vi "Main Dialog.vi"(11 "Process Path":path) -> ()   [LabVIEW 2020, in "Method Generation.lvlib" / "New API VI Dialog.lvclass"]
uses:
  New API VI Dialog.lvclass
  New API VI Dialog.lvclass/New API VI Dialog.ctl
  API VI Generator/API VI Generator.lvclass
panel:
  in  "Highlight changes?":bool=TRUE
  in  "Commit":bool
  in  "Cancel":bool
  in  "API Message":string
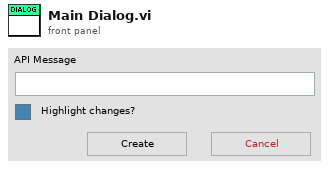
[diagram p1: front panel]
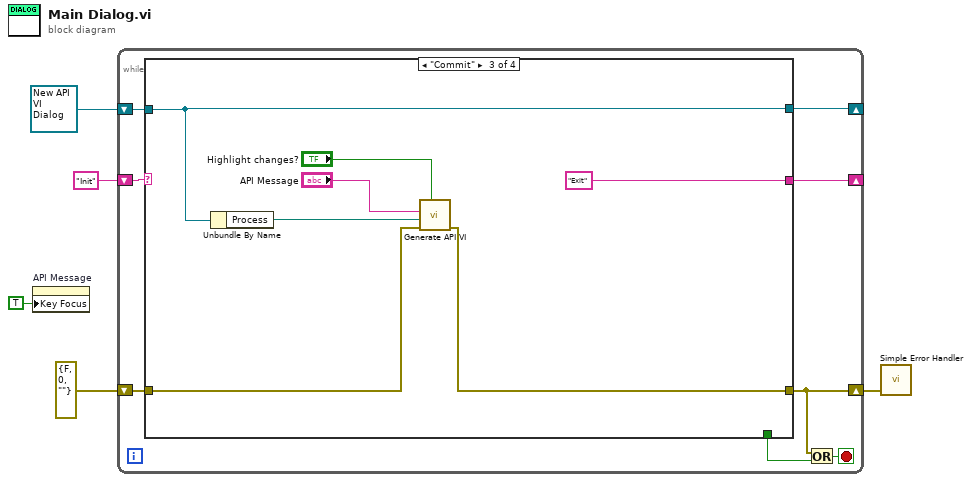
[diagram p0: block diagram]
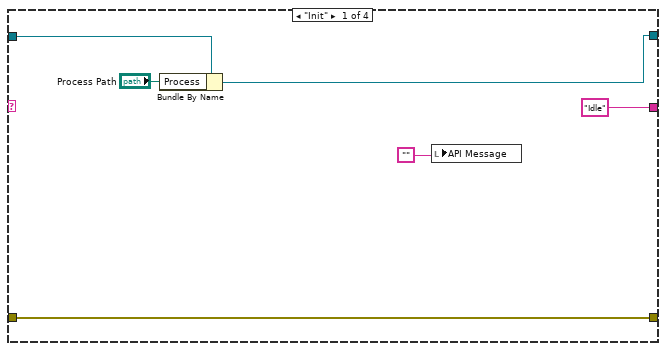
[diagram p2: hidden frame]
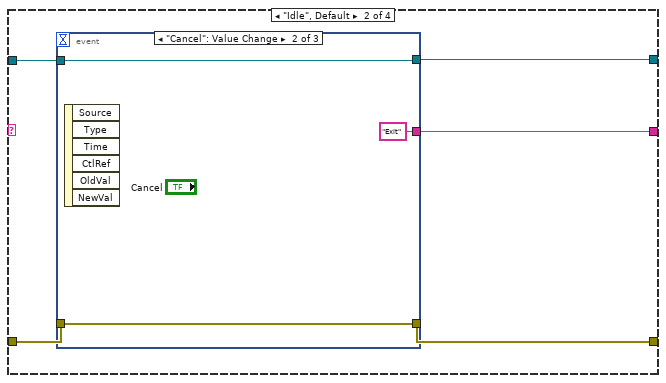
[diagram p3: hidden frame]
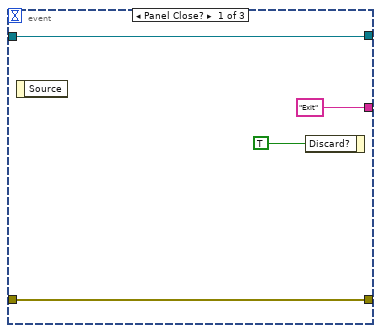
[diagram p4: hidden frame]
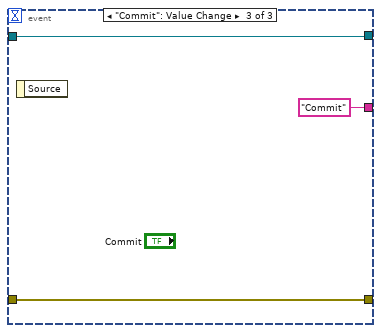
[diagram p5: hidden frame]
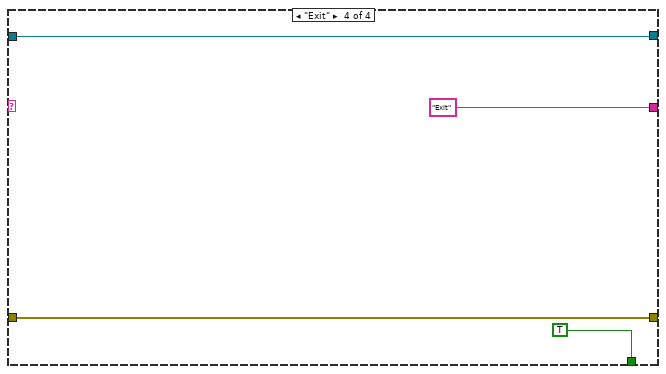
[diagram p6: hidden frame]
diagram:
  n1 = property on="API Message" class="Str"("Key Focus"=TRUE) -> ()  [unwired: 2 in, 2 out]
  n2 = while {
    shift-right: [w10] -> _
    shift-left: refnum<class "New API VI Dialog.lvclass"> refnum ("Method Generation.lvlib:New Getter Dialog.lvclass") -> [w11]
    shift-right: [w6] -> w2
    shift-left: errorcluster {"status"=FALSE, "code"=0, "source"=""} ("error in (no error)") -> [w12]
    shift-right: [w9] -> _
    shift-left: "Init" -> [w13]
    stop <- w7 stop-if-true
    n3 = case shown="\"Commit\"" w13 {
      tunnel: [w16 w24 w38 w44] -> w6
      tunnel: w12 -> [w16 w23 w37 w44]
      tunnel: w11 -> [w19 w22 w40 w45]
      tunnel: [w15 w21 w40 w45] -> w10
      tunnel: ["Idle" w20 "Exit" "Exit"] -> w9
      tunnel: [_ _ _ TRUE] -> w8
      frame "Init" {
        n4 = Bundle By Name(cluster=w19, "Process"="Process Path") -> (w15:refnum<class "New API VI Dialog.lvclass">)
        n5 = local write "API Message"("") -> ()
      }
      frame "Idle", Default {
        n6 = event shown="[1] \"Cancel\": Value Change" {
          selector: _ -> [_ _ _]
          dyn-events: _ -> [_ _ _]
          timeout: _ -> [_ _ _]
          tunnel: [w28 w30 w34] -> w24
          tunnel: w23 -> [w28 w30 w34]
          tunnel: w22 -> [w27 w31 w33]
          tunnel: [w27 w31 w33] -> w21
          tunnel: ["Exit" "Exit" "Commit"] -> w20
          event Panel Close? {
            n7 = event-data() -> ()  [unwired: 1 in, 1 out]
            n8 = event-data("Discard?"=TRUE) -> ()  [unwired: 1 in, 1 out]
          }
          event "Cancel": Value Change {
            n9 = event-data() -> ()  [unwired: 1 in, 6 out]
          }
          event "Commit": Value Change {
            n10 = event-data() -> ()  [unwired: 1 in, 1 out]
          }
        }
      }
      frame "Commit" {
        n11 = Unbundle By Name(w40) -> ("Process"=w39:path)
        n12 = call "Generate API VI.vi"("Highlight changes?"="Highlight changes?", "error in (no error)"=w37, "class path"=w39, "API Message"="API Message") -> ("error out"=w38:errorcluster)  [unwired: 7 in]
      }
      frame "Exit" {
      }
    }
    n13 = Or(x=w6, y=w8) -> (x .or. y?=w7:bool)
  }
  n14 = call <vilib>:"Simple Error Handler.vi"("error in (no error)"=w2) -> ()  [unwired: 4 in, 5 out]
